vi "Write Flags.vi"(8 "error in (no error)":errorcluster, 10 "Flags":u64, 11 "CIFfifo in":refnum<class "CIFfifo.lvclass">) -> (0 "error out":errorcluster, 3 "CIFfifo out":refnum<class "CIFfifo.lvclass">)   [LabVIEW 2021, in "CIFfifo.lvclass"]
uses:
  CIFfifo.lvclass
  CIFfifo.lvclass/CIFfifo.ctl
  ChannelCommon.lvlib
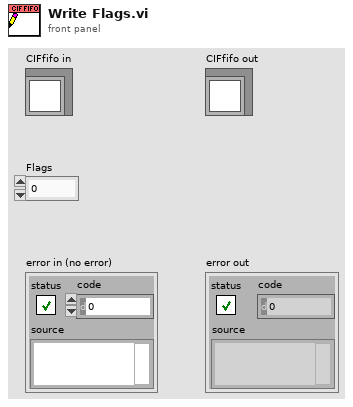
[diagram p1: front panel]
types:
  T1 = typedef "ChannelCommon.lvlib/FIFO Flags.ctl" = cluster{"Retry on Timeout":bool}
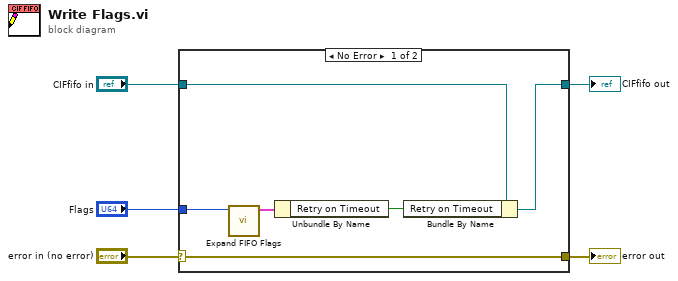
[diagram p0: block diagram]
diagram:
  n1 = case shown="No Error" "error in (no error)" {
    selector: "error in (no error)" -> [w11 w12]
    tunnel: [w11 w12] -> w4
    tunnel: [w9 w13] -> w2
    tunnel: "CIFfifo in" -> [w10 w13]
    tunnel: "Flags" -> [w8 _]
    frame No Error {
      n2 = call "Expand FIFO Flags.vi"("FIFO Flags"=w8) -> ("Flags"=w7:T1)  [unwired: 10 in]
      n3 = Unbundle By Name(w7) -> ("Retry on Timeout"=w6:bool)
      n4 = Bundle By Name(cluster=w10, "Retry on Timeout"=w6) -> (w9:refnum<class "CIFfifo.lvclass">)
    }
    frame Error {
    }
  }
  "error out" <- w4
  "CIFfifo out" <- w2
